vi "Handle Inlet Return.vi"(8 "error in":errorcluster, 11 "Log Session":T1) -> (0 "error out":errorcluster, 2 "Filter State":bool, 3 "Log Session Out":T1)   [LabVIEW 2018, in "Controller.lvlib" / "Controller.lvclass"]
uses:
  Controller.lvclass
  <userlib>/_Session Fwk/Typedefs/Session Handle.ctl
  <userlib>/_Session Fwk/Session - Root.lvclass
  <vilib>/DAQmx/read.llb/DAQmx Read (Digital 1D Bool NChan 1Samp 1Line).vi
  <vilib>/DAQmx/miscellaneous.llb/DAQmx Fill In Error Info.vi
  reusable/Session APIs/Session Log/System Log.lvclass
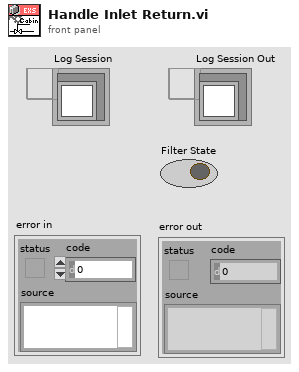
[diagram p1: front panel]
types:
  T1 = typedef "Session - Root.lvclass/Session Handle.ctl" = refnum<data-value>
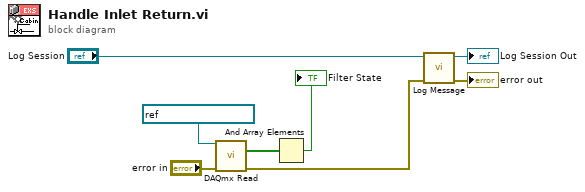
[diagram p0: block diagram]
diagram:
  n1 = call-poly <vilib>:"DAQmx Read.vi"("task/channels in"=refnum<k21> "Cabn Valve RTN", "error in"="error in") -> ("data"=w7:bool[], "error out"=w1:errorcluster)  [unwired: 11 in, 1 out]
  n2 = And Array Elements(Boolean array=w7) -> (logical AND=→"Filter State":bool)
  n3 = call "Log Message.vi"("error in"=w1, "session in"="Log Session") -> ("error out"=→"error out":errorcluster, "session out"=→"Log Session Out":T1)  [unwired: 8 in]
